vi "Get all devices core info.vi"() -> (0 "Array":cluster{"String":string, i32}[](array[cluster]), 1 "Array 2":cluster{"String":string, i32}[](array[cluster]), 2 "data":string[][](array[string]), 3 "> Name, devtype, ip, dev comm port, class, location for all devices>":string[][](array[string]))   [LabVIEW 2020]
uses:
  Shared/MySQL/Preset Query Enum.ctl
  <userlib>/_OpenG.lib/array/array.llb/Remove Duplicates from 1D Array (String)__ogtk.vi
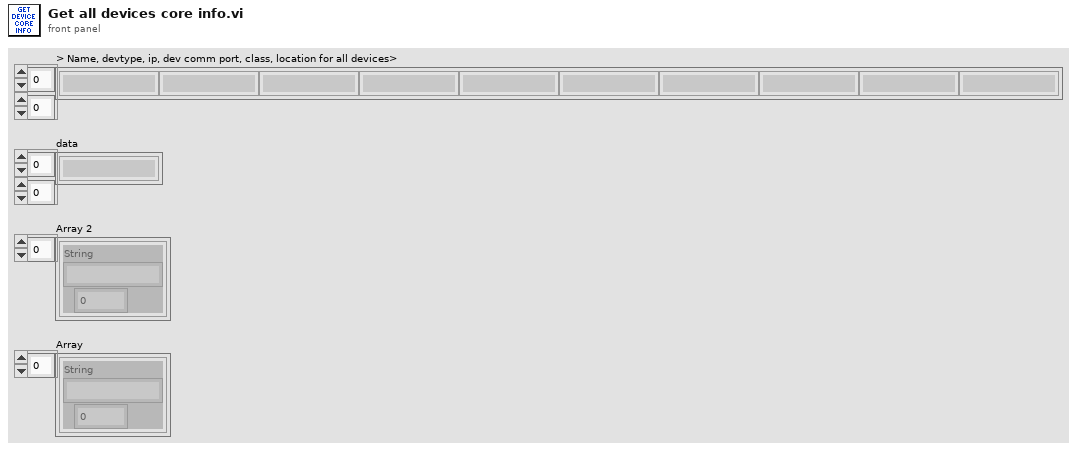
[diagram p1: front panel]
types:
  T1 = typedef "Preset Query Enum.ctl" = enum16{"Get Locations", "Get all IPs and MACs", "Get classes", "Get expt variables to set at scanstart for particular device", "Get expt devices and variables with start values", "Get expt devices and variables (with data to get)", "Get expt devices with data to get", "Get Expt devices and GUIs", "Get all devices basic properties", "Get Virtual Devices Core Info", "Get Expt names", "Get experiment basic properties", "Get experiment alarm variables", "Get MC Ports", "Get device network comm port", "Get devicetype lvclass path", "Get basic device properties", "Get Init Order", "Get all setable variables of a device", "Get device variable aliases", "Get force values of all settable variables", "Get all variables of a devicetype", "Get all variables of a device", "Get plotter details", "Get Saved Scans", "Get Scan Info", "GetGeneralGUIs", "Get expt for plotter", "Get plotter IDs from expt", "Get all devices", "Get all Virtual Devices", "Get all aliases", "Get variable and device info for Virtual Device", "GetItemLocatorIP", "Get IPs for GUIs", "Get DeviceType from Device", "GetLocalPortRange", "GetDevicePresetVariables", "Get Device Configuration", "GetAllPresetNames", "GetAllConfigurationNames", "GetPresetDeviceNames", "GetDeviceAliases", "GetDevicesOfClass"}
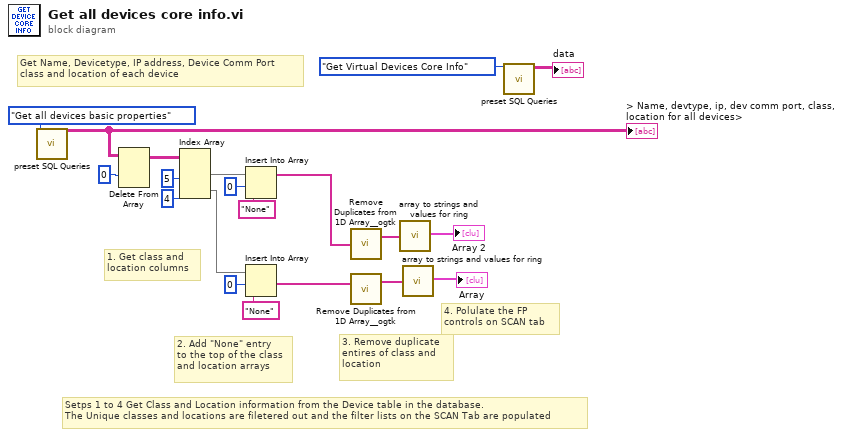
[diagram p0: block diagram]
diagram:
  # "Get Name, Devicetype, IP address, Device Comm Port\nclass and location of each device"
  # "4. Polulate the FP\ncontrols on SCAN tab"
  # "3. Remove duplicate \nentires of class and\nlocation"
  # "2. Add \"None\" entry\nto the top of the class\nand location arrays"
  # "1. Get class and \nlocation columns"
  # "Setps 1 to 4 Get Class and Location information from the Device table in the database.\nThe Unique classes and locations are filetered out and the filter lists on the SCAN Tab are populated"
  n1 = call "preset SQL Queries.vi"("Preset Query"=Preset_Query_Enum."Get all devices basic properties") -> ("data"=w3:string[][])  [unwired: 8 in, 2 out]
  "> Name, devtype, ip, dev comm port, class, location for all devices>" <- w3
  n2 = Delete From Array(array=w3, index (row)=0) -> (array with subset deleted=w12:string[][])  [unwired: 2 in, 1 out]
  n3 = Index Array(array=w12, index (col) #1=5 ("disabled index (col)"), index (col) #2=4 ("index (col)")) -> (element #1=w13:string[], element #2=w18:string[])  [unwired: 2 in]
  n4 = Insert Into Array(array=w13, index=0, new element="None" ("new element/subarray")) -> (w4:string[])
  n5 = Insert Into Array(array=w18, index=0, new element="None" ("new element/subarray")) -> (w6:string[])
  n6 = call-poly <userlib>:"Remove Duplicates from 1D Array__ogtk.vi"("Input Array"=w4) -> ("Output Array"=w5:string[])  [unwired: 1 out]
  n7 = call-poly <userlib>:"Remove Duplicates from 1D Array__ogtk.vi"("Input Array"=w6) -> ("Output Array"=w7:string[])  [unwired: 1 out]
  n8 = call "array to strings and values for ring.vi"("list of variables"=w5) -> ("Array"=→"Array 2":cluster{"String":string, i32}[])
  n9 = call "array to strings and values for ring.vi"("list of variables"=w7) -> ("Array"=→"Array":cluster{"String":string, i32}[])
  n10 = call "preset SQL Queries.vi"("Preset Query"=Preset_Query_Enum."Get Virtual Devices Core Info") -> ("data"=→"data":string[][])  [unwired: 8 in, 2 out]
